vi "RunOperation.vi"(10 "Inputs":string[](array[string]), 11 "DiscoverTestCases in":refnum<class "DiscoverTestCases.lvclass">) -> (1 "Output/Failure":string, 2 "CLI Process Return Code":i32, 3 "DiscoverTestCases out":refnum<class "DiscoverTestCases.lvclass">)   [LabVIEW 2027, in "DiscoverTestCases.lvclass"]
uses:
  DiscoverTestCases.lvclass
  DiscoverTestCases.lvclass/DiscoverTestCases.ctl
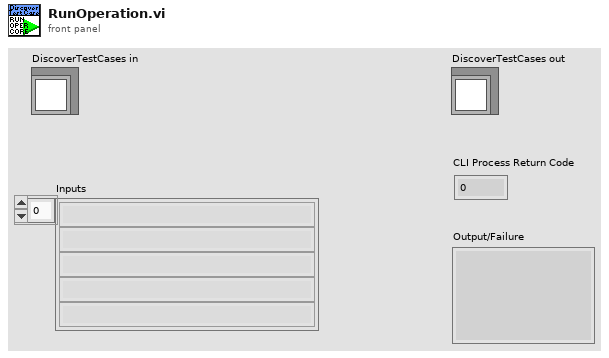
[diagram p1: front panel]
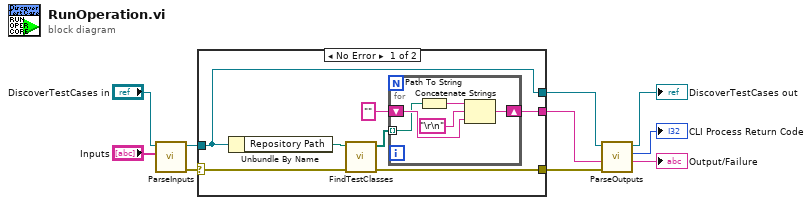
[diagram p0: block diagram]
diagram:
  n1 = call "ParseInputs.vi"("Inputs"="Inputs", "DiscoverTestCases in"="DiscoverTestCases in") -> ("error out"=w8:errorcluster, "DiscoverTestCases out"=w9:refnum<class "DiscoverTestCases.lvclass">)  [unwired: 8 in]
  n2 = case shown="No Error" w8 {
    selector: w8 -> [w15 w23]
    tunnel: [w13 w24] -> w6
    tunnel: w9 -> [w13 w24]
    tunnel: [w14 _] -> w1
    tunnel: [w11 w23] -> w2
    frame No Error {
      n3 = Unbundle By Name(w13) -> ("Repository Path"=w17:path)
      n4 = call "FindTestClasses.vi"("error in (no error)"=w15, "repository file path"=w17) -> ("error out"=w11:errorcluster, "Test Classes"=w16:path[])  [unwired: 8 in]
      n5 = for {
        tunnel: w16 -> [w20] mode=indexing
        shift-right: [w21] -> w14
        shift-left: "" -> [w22]
        n6 = Path To String(path=w20) -> (string=w19:string)
        n7 = Concatenate Strings(w19, "\r\n", w22) -> (w21:string)
      }
    }
    frame Error {
    }
  }
  n8 = call "ParseOutputs.vi"("error in (no error)"=w2, "Operation Output/Error In"=w1, "DiscoverTestCases in"=w6) -> ("Operation Output/Error Out"=→"Output/Failure":string, "CLI Process Return Code"=→"CLI Process Return Code":i32, "DiscoverTestCases out"=→"DiscoverTestCases out":refnum<class "DiscoverTestCases.lvclass">)  [unwired: 5 in, 1 out]
